vi "saveAnalyzerDataToTDMS.vi"(8 "ErrorIn":errorcluster, 11 "QueuesIn":T1) -> (0 "ErrorOut":errorcluster, 3 "QueuesOut":T1)   [LabVIEW 2019]
uses:
  utilities/Queues.ctl
  GUIVIs/GUIOutput.ctl
  MobileAnalyzer/mainVIs/analyzeAccelerationDataVIs/AnalyzedVibrationsData.ctl
  MobileAnalyzer/mainVIs/analyzeAccelerationDataVIs/AccelerationDataFrames.ctl
  MobileAnalyzer/mainVIs/analyzeAccelerationDataVIs/calculateFaultIndicatorsVIs/FaultDetections.ctl
  MobileAnalyzer/mainVIs/analyzeAccelerationDataVIs/calculateFaultIndicatorsVIs/ParameterFaultDetection.ctl
  MobileAnalyzer/mainVIs/analyzeAccelerationDataVIs/calculateFaultIndicatorsVIs/FaultParameter.ctl
  MobileAnalyzer/mainVIs/analyzeAccelerationDataVIs/calculateFaultIndicatorsVIs/FrequencyFaultDetection.ctl
  MobileAnalyzer/mainVIs/analyzeAccelerationDataVIs/calculateFaultIndicatorsVIs/OrdersFaultDetection.ctl
  masterVIs/Command.ctl
  MobileAnalyzer/mainVIs/TDMSmanagerVIs/TDMSAnalyzerData.ctl
  MobileAnalyzer/mainVIs/TDMSmanagerVIs/TDMSAnalyzerDataType.ctl
  saveAnalyzerDataToTDMSVIs/SignalDataToSave.ctl
  saveAnalyzerDataToTDMSVIs/saveAccelerationTimeDataToTDMSState.ctl
  masterVIs/Thread.ctl
panel:
  in  "AnalysisDataTDMS":refnum<k34>
  in  "Stop":bool=TRUE
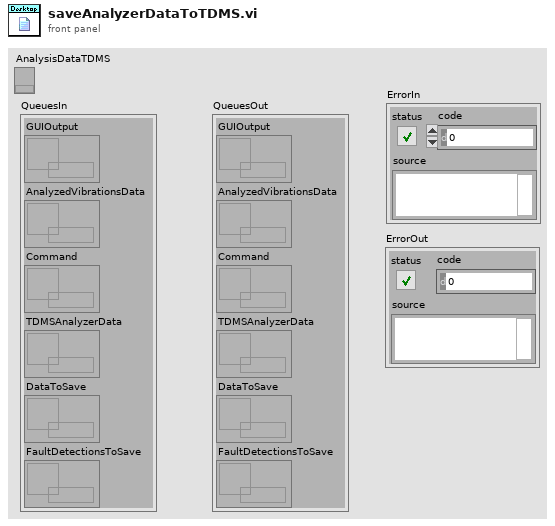
[diagram p1: front panel]
types:
  T1 = typedef "Queues.ctl" = cluster{"GUIOutput":refnum<queue>, "AnalyzedVibrationsData":refnum<queue>, "Command":refnum<queue>, "TDMSAnalyzerData":refnum<queue>, "DataToSave":refnum<queue>, "FaultDetectionsToSave":refnum<queue>}
  T2 = typedef "Thread.ctl" = enum16{"GUI", "communicateWithAnalyzer", "saveDataToTDMS"}
  T3 = typedef "saveAccelerationTimeDataToTDMSState.ctl" = enum16{"Idle", "Init", "Save to TDMS", "End"}
  T4 = typedef "Command.ctl" = enum16{"None", "Connect", "Start", "Stop", "RestartAnalyzer", "Exit", "OpenDataFile", "CanBegin", "FileToSaveSettings", "AnalyzerSettings", "DownloadDataDialog", "DownloadData", "DeleteData", "SendAnalysisData"}
  T5 = enum16{"open", "open or create", "create or replace", "create", "open (read-only)"}
  T6 = typedef "DesktopAppSettings.ctl" = cluster{"MobileAnalyzer IP":string, "Network Stream Timeout Code":i32, "Endpoint Destroyed Code":i32, "Save to file?":bool, "All threads":T2[], "Connected":bool, "SaveSignalsDir":path, "SaveAnalysisOnPC?":bool, "AnalysisSettings":T7}
  T7 = typedef "AnalysisSettings.ctl" = cluster{"Fault Thresholds":T8, "Analysis series name":string, "Save data analysis?":bool, "F-Band Size":i32, "OrderAnalysis?":bool, "Accelerometer":T10, "fs [Hz]":dbl, "Pulse per revolution":u16, "FFT-Parameters":cluster{"averaging mode":enum16{"No averaging", "Vector averaging", "RMS averaging", "Peak hold"}, "weighting mode":enum16{"Linear", "Exponential"}, "number of averages":u32}, "O-WindowPowerSpectrum":u32, "O-SpectrumAveraging":enum16{"No averaging", "Vector averaging", "RMS averaging", "Peak hold"}, "O-MaxOrder":dbl, "O-Resolution":dbl, "O-BandSize":dbl, "FrameLength [s]":dbl, "Aq.FrameLength [ms]":i64, "FilterOrder":i32, "Sensitivity [V/g]":dbl[]}
  T8 = typedef "Thresholds.ctl" = cluster{"Parameters labels":T9[], "Parameters thresholds":dbl[], "Freqs and thresholds":dbl[][], "Orders and thresholds":dbl[][]}
  T9 = typedef "FaultParameter.ctl" = enum16{"Kurtosis", "RMS", "Crest factor"}
  T10 = typedef "Accelerometer.ctl" = enum16{"None", "MPU6050", "MMA7351"}
  T11 = typedef "SignalDataToSave.ctl" = cluster{"Tacho signal":waveform(dbl), "AccelerationData":waveform(dbl)[]}
  T12 = typedef "FaultDetections.ctl" = cluster{"Parameters fault detection":T13[], "Frequencies fault detection":T14[], "Orders fault detection":T15[]}
  T13 = typedef "ParameterFaultDetection.ctl" = cluster{"Axes Values":dbl[], "Axes Fault Detection":bool[], "Parameter Label":T9}
  T14 = typedef "FrequencyFaultDetection.ctl" = cluster{"Axes Values":dbl[], "Axes Fault Detection":bool[], "Frequency":dbl}
  T15 = typedef "OrdersFaultDetection.ctl" = cluster{"Order":dbl, "Axes Fault Detection":bool[], "Axes Values":dbl[]}
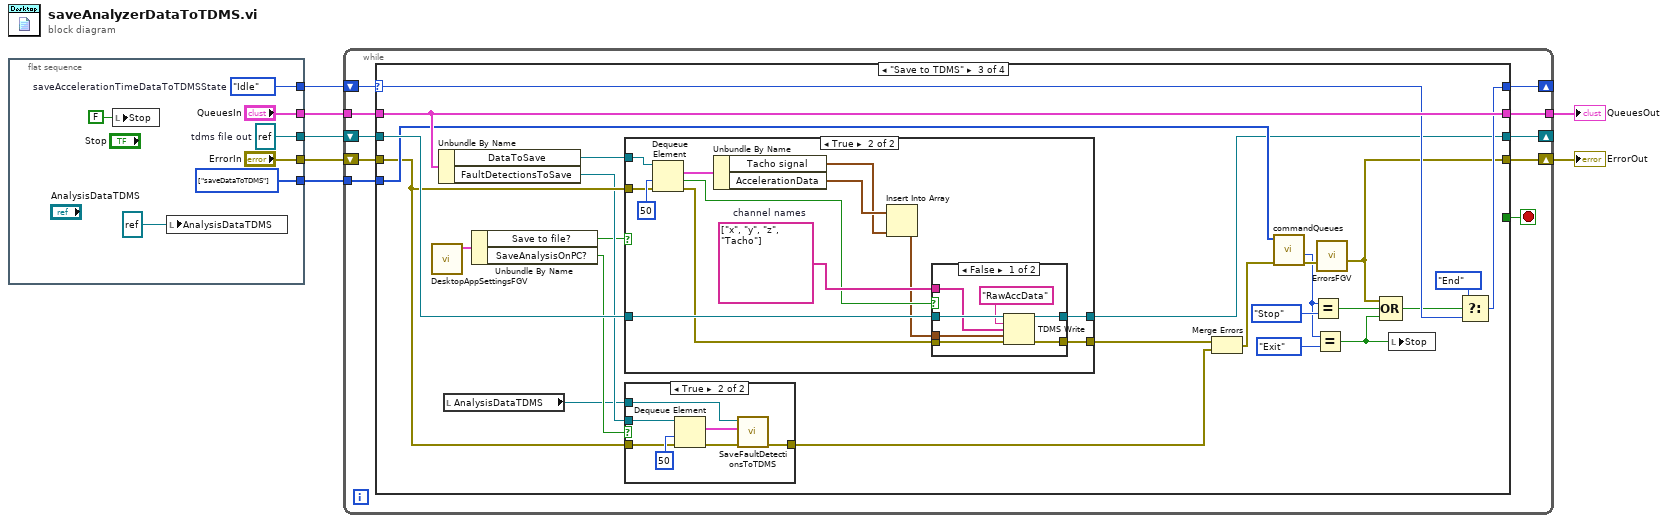
[diagram p0: block diagram]
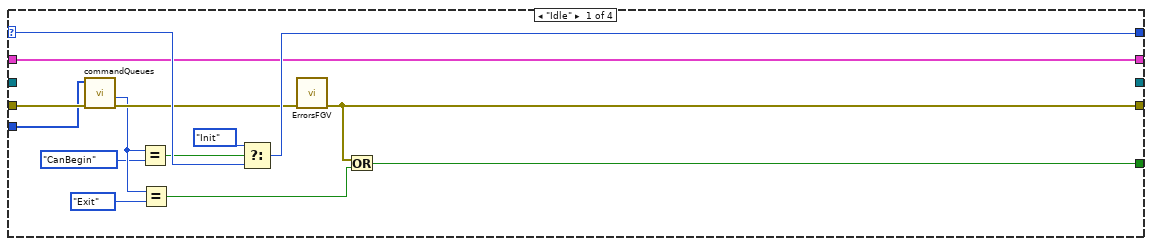
[diagram p2: hidden frame]
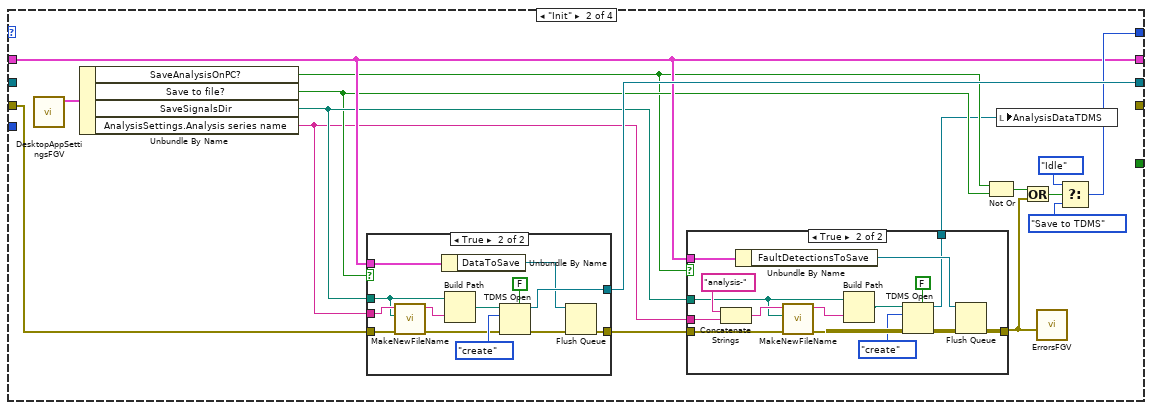
[diagram p3: hidden frame]
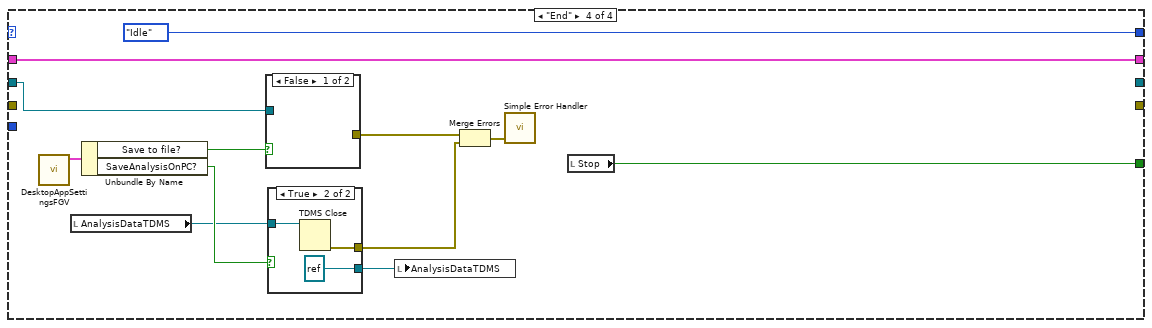
[diagram p9: hidden frame]
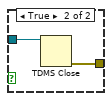
[diagram p11: hidden frame]
diagram:
  n1 = flat-sequence {
    tunnel: [w14] -> w7
    tunnel: ["ErrorIn"] -> w6
    tunnel: [w12] -> w1
    tunnel: ["QueuesIn"] -> w4
    tunnel: [w9] -> w2
    frame #0 {
      w9 = T2[] [enum."saveDataToTDMS"] items=["GUI", "communicateWithAnalyzer", "saveDataToTDMS"] ("Threads")
      w12 = refnum<k34> refnum  # tdms file out
      w14 = saveAccelerationTimeDataToTDMSState."Idle"  # saveAccelerationTimeDataToTDMSState
      n2 = local write "Stop"(FALSE ("Stop")) -> ()
      n3 = local write "AnalysisDataTDMS"(refnum<k34> refnum ("AnalysisDataTDMS")) -> ()
    }
  }
  n4 = while {
    shift-right: [w20] -> _
    shift-left: w7 -> [w24]
    tunnel: w4 -> [w23]
    shift-right: [w17] -> w5
    shift-left: w6 -> [w22]
    tunnel: [w21] -> w3
    shift-right: [w19] -> _
    shift-left: w1 -> [w18]
    tunnel: w2 -> [w15]
    stop <- w16 stop-if-true
    n5 = case shown="\"Save to TDMS\"" w24 {
      selector: w24 -> [w38 _ w107 _]
      tunnel: w23 -> [w35 w47 w109 w152]
      tunnel: w22 -> [w29 w48 w93 _]
      tunnel: [w35 w47 w109 w152] -> w21
      tunnel: [w31 _ w86 _] -> w17
      tunnel: [w36 _ _ w151] -> w16
      tunnel: [w37 w50 w105 saveAccelerationTimeDataToTDMSState."Idle" ("saveAccelerationTimeDataToTDMSState")] -> w20
      tunnel: [_ w54 w96 _] -> w19
      tunnel: w18 -> [_ _ w108 w146]
      tunnel: w15 -> [w26 _ w98 _]
      frame "Idle" {
        n6 = call "commandQueues.vi"("ErrorIn"=w29, "Threads"=w26) -> ("ErrorOut"=w28:errorcluster, "CommandOut"=w27:T4)  [unwired: 8 in]
        n7 = Equal?(x=w27, y=Command."CanBegin") -> (x = y?=w33:bool)
        n8 = Equal?(x=w27, y=Command."Exit") -> (x = y?=w30:bool)
        n9 = Select(t=saveAccelerationTimeDataToTDMSState."Init", s=w33, f=w38) -> (s? t:f=w37:T3)
        n10 = call "ErrorsFGV.vi"("CriticalErrorIn"=w28) -> ("CriticalErrorOut"=w31:errorcluster)  [unwired: 7 in, 3 out]
        n11 = Or(x=w31, y=w30) -> (x .or. y?=w36:bool)
      }
      frame "Init" {
        n12 = call "DesktopAppSettingsFGV.vi"() -> ("DesktopAppSettingsOut"=w49:T6)  [unwired: 11 in]
        n13 = Unbundle By Name(w49) -> ("SaveAnalysisOnPC?"=w43:bool, "Save to file?"=w44:bool, "SaveSignalsDir"=w46:path, "AnalysisSettings.Analysis series name"=w39:string)
        n14 = case shown="True" w44 {
          tunnel: w48 -> [w71 w76]
          tunnel: [w71 w78] -> w45
          tunnel: [_ w82] -> w54
          tunnel: w47 -> [_ w81]
          tunnel: w39 -> [_ w74]
          tunnel: w46 -> [_ w73]
          frame False {
          }
          frame True {
            n15 = call "MakeNewFileName.vi"("ErrorIn"=w76, "Dir"=w73, "SeriesString"=w74) -> ("ErrorOut"=w75:errorcluster, "NewFileName"=w72:string)  [unwired: 7 in]
            n16 = Unbundle By Name(w81) -> ("DataToSave"=w80:refnum<queue>)
            n17 = Build Path(base path=w73, name or relative path=w72) -> (appended path=w77:path)
            n18 = TDMS Open(5:FALSE ("create index file? (T)"), 8:w75, 10:T5."create" ("operation (0:open)"), 11:w77) -> (0:w79:errorcluster, 3:w82:refnum<k34>)  [unwired: 3 in]
            n19 = Flush Queue(queue=w80, error in (no error)=w79) -> (error out=w78:errorcluster)  [unwired: 2 out]
          }
        }
        n20 = case shown="True" w43 {
          tunnel: w47 -> [_ w70]
          tunnel: w46 -> [_ w57]
          tunnel: w39 -> [_ w68]
          tunnel: w45 -> [w55 w60]
          tunnel: [w55 w63] -> w41
          tunnel: [_ w61] -> w40
          frame False {
          }
          frame True {
            n21 = Concatenate Strings("analysis-", w68) -> (w58:string)
            n22 = Unbundle By Name(w70) -> ("FaultDetectionsToSave"=w62:refnum<queue>)
            n23 = call "MakeNewFileName.vi"("ErrorIn"=w60, "Dir"=w57, "SeriesString"=w58) -> ("ErrorOut"=w59:errorcluster, "NewFileName"=w56:string)  [unwired: 7 in]
            n24 = Build Path(base path=w57, name or relative path=w56) -> (appended path=w66:path)
            n25 = TDMS Open(5:FALSE ("create index file? (T)"), 8:w59, 10:T5."create" ("operation (0:open)"), 11:w66) -> (0:w64:errorcluster, 3:w61:refnum<k34>)  [unwired: 3 in]
            n26 = Flush Queue(queue=w62, error in (no error)=w64) -> (error out=w63:errorcluster)  [unwired: 2 out]
          }
        }
        n27 = Not Or(1:w44, 2:w43) -> (0:w42:bool)
        n28 = local write "AnalysisDataTDMS"(w40) -> ()
        n29 = Or(x=w42, y=w41) -> (x .or. y?=w53:bool)
        n30 = call "ErrorsFGV.vi"("InternalErrorIn"=w41) -> ()  [unwired: 7 in, 4 out]
        n31 = Select(t=saveAccelerationTimeDataToTDMSState."Idle", s=w53, f=saveAccelerationTimeDataToTDMSState."Save to TDMS" ("saveAccelerationTimeDataToTDMSState")) -> (s? t:f=w50:T3)
      }
      frame "Save to TDMS" {
        n32 = call "DesktopAppSettingsFGV.vi"() -> ("DesktopAppSettingsOut"=w89:T6)  [unwired: 11 in]
        n33 = Unbundle By Name(w109) -> ("DataToSave"=w94:refnum<queue>, "FaultDetectionsToSave"=w92:refnum<queue>)
        n34 = local read "AnalysisDataTDMS"() -> (w85:refnum<k34>)
        n35 = Unbundle By Name(w89) -> ("Save to file?"=w88:bool, "SaveAnalysisOnPC?"=w87:bool)
        n36 = case shown="True" w88 {
          tunnel: w108 -> [w119 w131]
          tunnel: [w119 w121] -> w96
          tunnel: [w118 w120] -> w95
          tunnel: w94 -> [_ w126]
          tunnel: w93 -> [w118 w125]
          frame False {
          }
          frame True {
            w128 = string[] ["x", "y", "z", "Tacho"]  # channel names
            n37 = Dequeue Element(queue=w126, timeout in ms (-1)=50, error in (no error)=w125) -> (element=w129:T11, timed out?=w127:bool, error out=w130:errorcluster)  [unwired: 1 out]
            n38 = Unbundle By Name(w129) -> ("Tacho signal"=w123:waveform(dbl), "AccelerationData"=w124:waveform(dbl)[])
            n39 = Insert Into Array(array=w124, new element=w123) -> (w122:waveform(dbl)[])  [unwired: 1 in]
            n40 = case shown="False" w127 {
              tunnel: w131 -> [w139 w141]
              tunnel: w130 -> [w138 w140]
              tunnel: [w136 w140] -> w120
              tunnel: [w135 w141] -> w121
              tunnel: w122 -> [w134 _]
              tunnel: w128 -> [w133 _]
              frame False {
                n41 = TDMS Write(0:w139, 5:"RawAccData" ("group name in (Untitled)"), 7:w133, 9:w134, 11:w138) -> (4:w135:refnum<k34>, 15:w136:errorcluster)  [unwired: 1 in, 2 out]
              }
              frame True {
              }
            }
          }
        }
        n42 = case shown="True" w87 {
          tunnel: w93 -> [w110 w116]
          tunnel: w92 -> [_ w115]
          tunnel: w85 -> [_ w114]
          tunnel: [w110 w111] -> w90
          frame False {
          }
          frame True {
            n43 = Dequeue Element(queue=w115, timeout in ms (-1)=50, error in (no error)=w116) -> (element=w113:T12, error out=w112:errorcluster)  [unwired: 2 out]
            n44 = call "SaveFaultDetectionsToTDMS.vi"("error in (no error)"=w112, "Fault detections"=w113, "Refnum in"=w114) -> ("error out"=w111:errorcluster)  [unwired: 7 in, 1 out]
          }
        }
        n45 = Merge Errors(w95, w90) -> (w91:errorcluster)
        n46 = call "commandQueues.vi"("ErrorIn"=w91, "Threads"=w98) -> ("ErrorOut"=w99:errorcluster, "CommandOut"=w97:T4)  [unwired: 8 in]
        n47 = Equal?(x=w97, y=Command."Stop") -> (x = y?=w103:bool)
        n48 = Equal?(x=w97, y=Command."Exit") -> (x = y?=w100:bool)
        n49 = call "ErrorsFGV.vi"("InternalErrorIn"=w99) -> ("InternalErrorOut"=w86:errorcluster)  [unwired: 7 in, 3 out]
        n50 = Compound Arithmetic op=OR(w86, w103, w100) -> (w101:bool)
        n51 = local write "Stop"(w100) -> ()
        n52 = Select(t=saveAccelerationTimeDataToTDMSState."End", s=w101, f=w107) -> (s? t:f=w105:T3)
      }
      frame "End" {
        n53 = call "DesktopAppSettingsFGV.vi"() -> ("DesktopAppSettingsOut"=w148:T6)  [unwired: 11 in]
        n54 = local read "AnalysisDataTDMS"() -> (w144:refnum<k34>)
        n55 = Unbundle By Name(w148) -> ("Save to file?"=w147:bool, "SaveAnalysisOnPC?"=w145:bool)
        n56 = case shown="False" w147 {
          tunnel: [_ w158] -> w150
          tunnel: w146 -> [_ w157]
          frame False {
          }
          frame True {
            n57 = TDMS Close(11:w157) -> (0:w158:errorcluster)  [unwired: 1 in, 1 out]
          }
        }
        n58 = case shown="True" w145 {
          tunnel: [_ w156] -> w143
          tunnel: w144 -> [_ w155]
          tunnel: [_ refnum<k34> refnum ("AnalysisDataTDMS")] -> w142
          frame False {
          }
          frame True {
            n59 = TDMS Close(11:w155) -> (0:w156:errorcluster)  [unwired: 1 in, 1 out]
          }
        }
        n60 = local write "AnalysisDataTDMS"(w142) -> ()
        n61 = Merge Errors(w150, w143) -> (w149:errorcluster)
        n62 = call <vilib>:"Simple Error Handler.vi"("error in (no error)"=w149) -> ()  [unwired: 4 in, 5 out]
        n63 = local read "Stop"() -> (w151:bool)
      }
    }
  }
  "ErrorOut" <- w5
  "QueuesOut" <- w3
